vi "DestroySelfReference.vi"(8 "error in (no error)":errorcluster, 11 "Subsystem":refnum<class "DAQmx(AI).lvclass">) -> (0 "error out":errorcluster, 3 "Subsystem out":refnum<class "DAQmx(AI).lvclass">)   [LabVIEW 2013, in "DAQmx(AI).lvclass"]
doc: "JKI State Machine Objects (SMO) 1.0.0.5\nJKI - JKI\nCopyright (c) 2016, JKI"
uses:
  DAQmx(AI).lvclass
  <vilib>/JKI/JKI SMO/SMO/SMO.lvclass
  DAQmx(AI).lvclass/DAQmx(AI).ctl
panel:
  # "For instructions on how to use the JKI State Machine Objects, examples and video tutorials, visit:\nhttp://jki.net/state-machine-objects/\n\nJKI State Machine Objects™\nhttp://jki.net/state-machine-objects/\nCopyright (C) 2005-2015, JKI <info@jki.net>\nALL RIGHTS RESERVED"
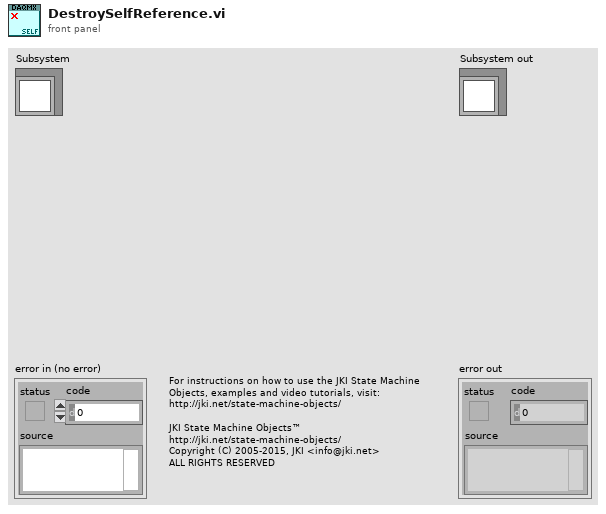
[diagram p1: front panel]
types:
  T1 = typedef "DAQmx(AI).lvclass/PrivateData--Ref.ctl" = refnum<data-value>
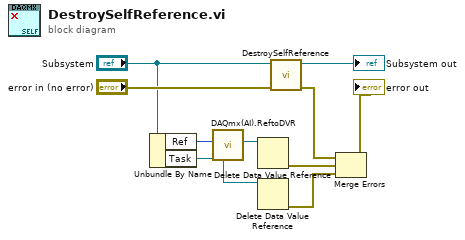
[diagram p0: block diagram]
diagram:
  n1 = Unbundle By Name("Subsystem") -> ("Ref"=w4:u32, "Task"=w2:refnum<data-value>)
  n2 = call "DAQmx(AI).ReftoDVR.vi"("Ref"=w4) -> ("Ref"=w3:T1)  [unwired: 10 in]
  n3 = Delete Data Value Reference(data value reference=w3) -> (error out=w7:errorcluster)  [unwired: 1 in, 1 out]
  n4 = Delete Data Value Reference(data value reference=w2) -> (error out=w1:errorcluster)  [unwired: 1 in, 1 out]
  n5 = call-parent "DestroySelfReference.vi"("error in (no error)"="error in (no error)", "SMO"="Subsystem") -> ("error out"=w6:errorcluster, "SMO out"=→"Subsystem out":refnum<class "DAQmx(AI).lvclass">)  [unwired: 8 in]
  n6 = Merge Errors(w6, w7, w1) -> (→"error out":errorcluster)
